vi "F3Machine_1.vi"   [LabVIEW 2011]
uses:
  API/API DYM.lvlib
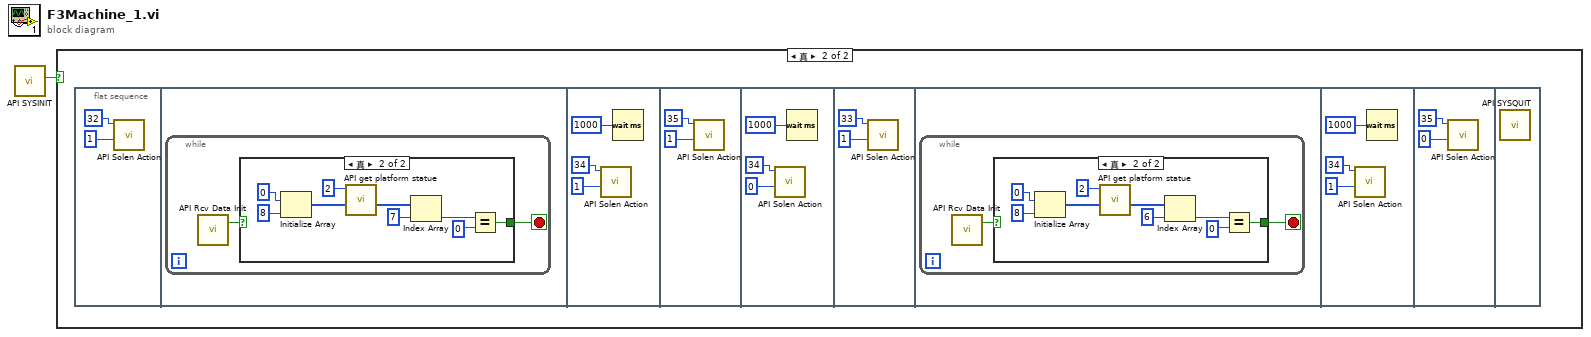
[diagram p0: block diagram]
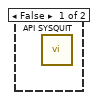
[diagram p2: hidden frame]
diagram:
  n1 = call "API SYSINIT.vi"() -> ("SYSINIT return value"=w1:bool)  [unwired: 11 in]
  n2 = case shown="真" w1 {
    frame False {
      n3 = call "API SYSQUIT.vi"() -> ()  [unwired: 12 in]
    }
    frame True {
      n4 = flat-sequence {
        frame #0 {
          n5 = call "API Solen Action.vi"("statue"=1, "solenNum"=32) -> ()  [unwired: 9 in, 1 out]
        }
        frame #1 {
          n6 = while {
            stop <- w4 stop-if-true
            n7 = call "API Rcv Data Init.vi"() -> ("RTV"=w5:bool)  [unwired: 2 in, 1 out]
            n8 = case shown="真" w5 {
              selector: w5 -> [w6 _]
              tunnel: [w6 w7] -> w4
              frame False {
              }
              frame True {
                n9 = Initialize Array(0 ("元素"), 8 ("维数大小")) -> (w12:i32[])
                n10 = call "API get platform statue.vi"("platformStatue input"=w12, "PlatformNum"=2) -> ("platformStatue output"=w11:i32[])  [unwired: 8 in, 1 out]
                n11 = Index Array(array=w11, index=7 ("索引")) -> (element=w9:i32)
                n12 = Equal?(x=w9, y=0) -> (x = y?=w7:bool)
              }
            }
          }
        }
        frame #2 {
          n13 = call "API Solen Action.vi"("statue"=1, "solenNum"=34) -> ()  [unwired: 9 in, 1 out]
          n14 = Wait (ms)(milliseconds to wait=u32 1000 ("等待时间（毫秒）")) -> ()  [unwired: 1 out]
        }
        frame #3 {
          n15 = call "API Solen Action.vi"("statue"=1, "solenNum"=35) -> ()  [unwired: 9 in, 1 out]
        }
        frame #4 {
          n16 = call "API Solen Action.vi"("statue"=0, "solenNum"=34) -> ()  [unwired: 9 in, 1 out]
          n17 = Wait (ms)(milliseconds to wait=u32 1000 ("等待时间（毫秒）")) -> ()  [unwired: 1 out]
        }
        frame #5 {
          n18 = call "API Solen Action.vi"("statue"=1, "solenNum"=33) -> ()  [unwired: 9 in, 1 out]
        }
        frame #6 {
          n19 = while {
            stop <- w26 stop-if-true
            n20 = call "API Rcv Data Init.vi"() -> ("RTV"=w27:bool)  [unwired: 2 in, 1 out]
            n21 = case shown="真" w27 {
              selector: w27 -> [w28 _]
              tunnel: [w28 w29] -> w26
              frame False {
              }
              frame True {
                n22 = Initialize Array(0 ("元素"), 8 ("维数大小")) -> (w34:i32[])
                n23 = call "API get platform statue.vi"("platformStatue input"=w34, "PlatformNum"=2) -> ("platformStatue output"=w33:i32[])  [unwired: 8 in, 1 out]
                n24 = Index Array(array=w33, index=6 ("索引")) -> (element=w31:i32)
                n25 = Equal?(x=w31, y=0) -> (x = y?=w29:bool)
              }
            }
          }
        }
        frame #7 {
          n26 = call "API Solen Action.vi"("statue"=1, "solenNum"=34) -> ()  [unwired: 9 in, 1 out]
          n27 = Wait (ms)(milliseconds to wait=u32 1000 ("等待时间（毫秒）")) -> ()  [unwired: 1 out]
        }
        frame #8 {
          n28 = call "API Solen Action.vi"("statue"=0, "solenNum"=35) -> ()  [unwired: 9 in, 1 out]
        }
        frame #9 {
          n29 = call "API SYSQUIT.vi"() -> ()  [unwired: 12 in]
        }
      }
    }
  }
